vi "RowColSelect.vi"(7 "HWSettings":T1={"Nr. of Columns"=1, "Nr. of Rows"=18, "OverSampling"=10, "Fetch Rate "=20, "Sampling Rate"=50000, "Nr. of BNC inputs"=3, "Sample Strip Length"=10} caption="Hardware Settingss", 9 "Row/Col Index":dbl, 10 "Row/Col Select":enum16{"Show single column", "Show single row"}(ring), 11 "DATA IN":dbl[](array[numeric])) -> (1 "DATA OUT":dbl[](array[numeric]))   [LabVIEW 2011]
uses:
  controls/General Hardware config.ctl
panel:
  # "Array"
  # "Acq. System"
  # "Other analog Input"
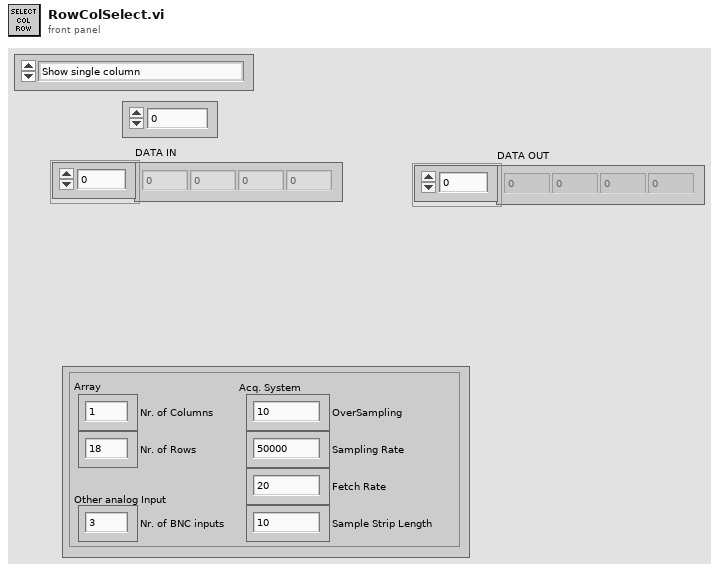
[diagram p1: front panel]
types:
  T1 = typedef "General Hardware config.ctl" = cluster{"Nr. of Columns":i32, "Nr. of Rows":i32, "OverSampling":i32, "Fetch Rate ":i32, "Sampling Rate":i32, "Nr. of BNC inputs":i32, "Sample Strip Length":i32}
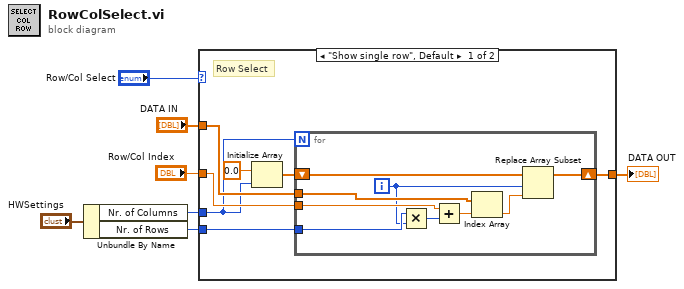
[diagram p0: block diagram]
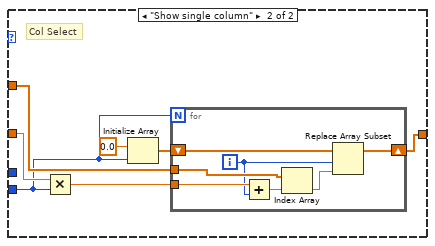
[diagram p2: hidden frame]
diagram:
  n1 = Unbundle By Name("HWSettings") -> ("Nr. of Columns"=w4:i32, "Nr. of Rows"=w3:i32)
  n2 = case shown="\"Show single row\", Default" "Row/Col Select" {
    tunnel: "DATA IN" -> [w13 w29]
    tunnel: "Row/Col Index" -> [w9 w28]
    tunnel: w4 -> [w8 _]
    tunnel: w3 -> [w10 w24]
    tunnel: [w12 w26] -> w2
    frame "Show single row", Default {
      # "Row Select"
      n3 = Initialize Array(0.0 ("element"), w8) -> (w11:dbl[])
      n4 = for {
        N: w8 -> [_]
        tunnel: w13 -> [w23]
        tunnel: w9 -> [w19]
        shift-right: [w20] -> w12
        shift-left: w11 -> [w22]
        tunnel: w10 -> [w18]
        i -> [w15]
        n5 = Multiply(x=w18, y=w15) -> (x*y=w17:i32)
        n6 = Add(x=w19, y=w17) -> (x+y=w16:dbl)
        n7 = Index Array(array=w23, index=w16) -> (element=w21:dbl)
        n8 = Replace Array Subset(array=w22, new element=w21, index=w15) -> (w20:dbl[])
      }
    }
    frame "Show single column" {
      # "Col Select"
      n9 = Multiply(x=w28, y=w24) -> (x*y=w27:dbl)
      n10 = Initialize Array(0.0 ("element"), w24) -> (w25:dbl[])
      n11 = for {
        N: w24 -> [_]
        tunnel: w29 -> [w37]
        tunnel: w27 -> [w36]
        shift-right: [w31] -> w26
        shift-left: w25 -> [w34]
        i -> [w33]
        n12 = Add(x=w36, y=w33) -> (x+y=w35:dbl)
        n13 = Index Array(array=w37, index=w35) -> (element=w32:dbl)
        n14 = Replace Array Subset(array=w34, new element=w32, index=w33) -> (w31:dbl[])
      }
    }
  }
  "DATA OUT" <- w2
